vi "stopBuildWorker.vi"(8 "error in (no error)":errorcluster, 11 "BuildWorker Basics in":refnum<class "BuildWorker Local.lvclass">) -> (0 "error out":errorcluster, 3 "BuildWorker Basics out":refnum<class "BuildWorker Local.lvclass">)   [LabVIEW 2017, in "BuildWorker Interface.lvlib" / "BuildWorker Local.lvclass"]
uses:
  BuildWorker Local.lvclass
  BuildWorker Local.lvclass/BuildWorker Local.ctl
  <vilib>/ActorFramework/Message Enqueuer/Message Enqueuer.lvclass/Message Enqueuer.ctl
  <vilib>/ActorFramework/Message Enqueuer/Enqueue.vi
  <vilib>/ActorFramework/Stop Msg/Stop Msg.lvclass
  C:/Program Files (x86)/National Instruments/LabVIEW 2017/vi.lib/ActorFramework/Message/Message.lvclass
  <vilib>/ActorFramework/Message Priority Queue/Priority Enqueue.vi
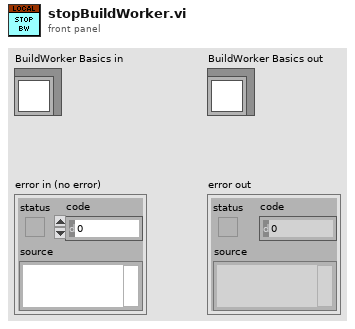
[diagram p1: front panel]
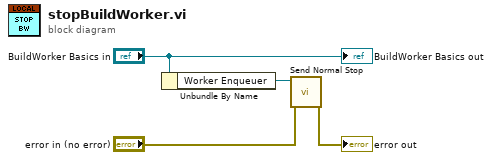
[diagram p0: block diagram]
diagram:
  n1 = Unbundle By Name("BuildWorker Basics in") -> ("Worker Enqueuer"=w3:refnum<class "Message Enqueuer.lvclass">)
  n2 = call <vilib>:"Send Normal Stop.vi"("error in (no error)"="error in (no error)", "Message Enqueuer"=w3) -> ("error out"=→"error out":errorcluster)  [unwired: 9 in]
  "BuildWorker Basics out" <- "BuildWorker Basics in"
